vi "Deposit.vi"(8 "file path":path, 9 "before match":string, 10 "after match":string) -> (2 "String":string)   [LabVIEW 2023]
uses:
  <vilib>/Utility/file.llb/Read Delimited Spreadsheet (string).vi
  <vilib>/Utility/file.llb/Write Delimited Spreadsheet (string).vi
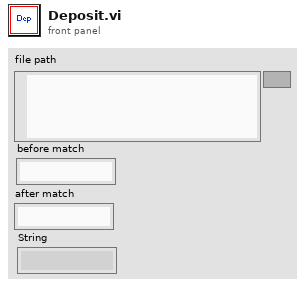
[diagram p1: front panel]
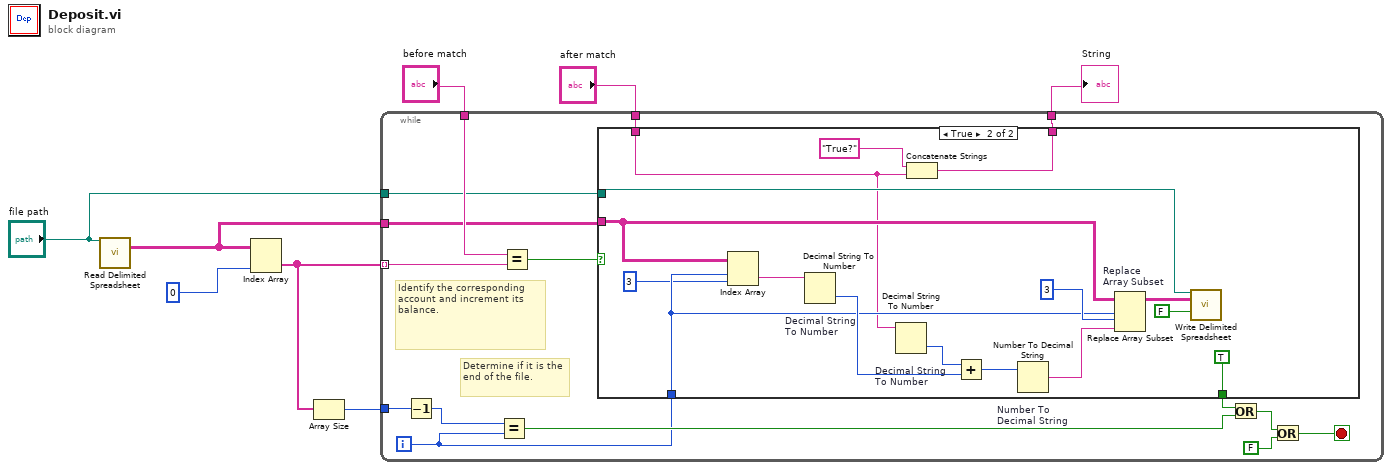
[diagram p0: block diagram]
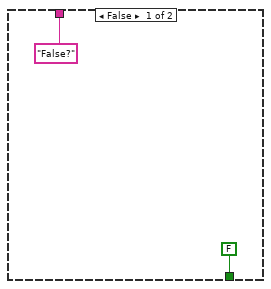
[diagram p2: hidden frame]
diagram:
  n1 = call-poly <vilib>:"Read Delimited Spreadsheet.vi"("file path (dialog if empty)"="file path") -> ("all rows"=w6:string[][])  [unwired: 9 in, 5 out]
  n2 = Index Array "Index Array"(array=w6, index (col)=0 ("index")) -> (element=w7:string[])  [unwired: 1 in]
  n3 = Array Size(array=w7) -> (size(s)=w8:i32)
  n4 = while {
    tunnel: w8 -> [w18]
    tunnel: w7 -> [w16] mode=indexing
    tunnel: "before match" -> [w15]
    tunnel: w6 -> [w12]
    tunnel: "file path" -> [w10]
    tunnel: "after match" -> [w11]
    tunnel: [w9] -> w1
    i -> [w13]
    stop <- w23 stop-if-true
    # "Determine if it is the end of the file."
    # "Identify the corresponding account and increment its balance."
    n5 = Decrement(x=w18) -> (x-1=w19:i32)
    n6 = Equal?(x=w19, y=w13) -> (x = y?=w17:bool)
    n7 = Equal?(x=w15, y=w16) -> (x = y?=w14:bool)
    n8 = case shown="True" w14 {
      tunnel: [FALSE TRUE] -> w20
      tunnel: w13 -> [_ w30]
      tunnel: w12 -> [_ w34]
      tunnel: w11 -> [_ w28]
      tunnel: w10 -> [_ w35]
      tunnel: ["False?" w26] -> w9
      frame False {
      }
      frame True {
        n9 = Index Array "Index Array"(array=w34, index (row)=w30, index (col)=3 ("disabled index (row)")) -> (element=w40:string)
        n10 = Decimal String To Number "Decimal String\nTo Number"(string=w40) -> (number=w38:i32)  [unwired: 2 in, 1 out]
        n11 = Decimal String To Number "Decimal String \nTo Number"(string=w28) -> (number=w39:i32)  [unwired: 2 in, 1 out]
        n12 = Concatenate Strings "Concatenate Strings"("True?", w28) -> (w26:string)
        n13 = Add(x=w39, y=w38) -> (x+y=w37:i32)
        n14 = Number To Decimal String "Number To \nDecimal String"(number=w37) -> (decimal integer string=w32:string)  [unwired: 1 in]
        n15 = Replace Array Subset "Replace \nArray Subset"(array=w34, new element=w32, index (row)=w30, index (col)=3 ("disabled index (col)")) -> (w31:string[][])
        n16 = call-poly <vilib>:"Write Delimited Spreadsheet.vi"("file path (dialog if empty)"=w35, "2D data"=w31, "append to file? (new file:F)"=FALSE) -> ()  [unwired: 11 in, 2 out]
      }
    }
    n17 = Or(x=w20, y=w17) -> (x .or. y?=w21:bool)
    n18 = Or(x=w21, y=FALSE) -> (x .or. y?=w23:bool)
  }
  "String" <- w1
